vi "read device registers.vi"() -> (4 "Sorted Device Names":string[](array[string]), 6 "All Registers":T1(array[cluster]), 8 "Camera Registers":T1(array[cluster]), 15 "Found Registers":bool)   [LabVIEW 2010]
uses:
  <vilib>/Utility/file.llb/Read From Spreadsheet File (I64).vi
  <vilib>/Utility/file.llb/Read From Spreadsheet File (string).vi
panel:
  out "All registers":T2(array[cluster])
  in  "Register":T3
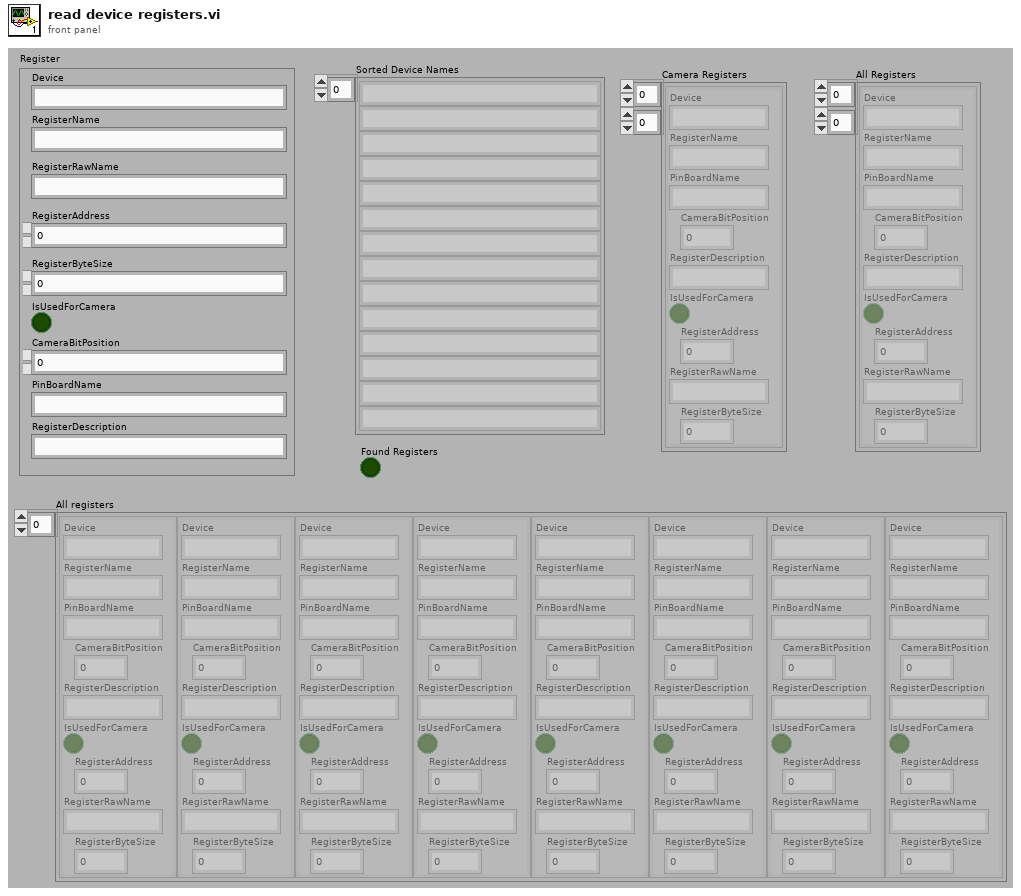
[diagram p1: front panel]
types:
  T1 = cluster{"Device":string, "RegisterName":string, "PinBoardName":string, "CameraBitPosition":i32, "RegisterDescription":string, "IsUsedForCamera":bool, "RegisterAddress":i32, "RegisterRawName":string, "RegisterByteSize":i32}[][]
  T2 = cluster{"Device":string, "RegisterName":string, "PinBoardName":string, "CameraBitPosition":i32, "RegisterDescription":string, "IsUsedForCamera":bool, "RegisterAddress":i32, "RegisterRawName":string, "RegisterByteSize":i32}[]
  T3 = cluster{"Device":string, "RegisterName":string, "PinBoardName":string, "CameraBitPosition":i32, "RegisterDescription":string, "IsUsedForCamera":bool, "RegisterAddress":i32, "RegisterRawName":string, "RegisterByteSize":i32}
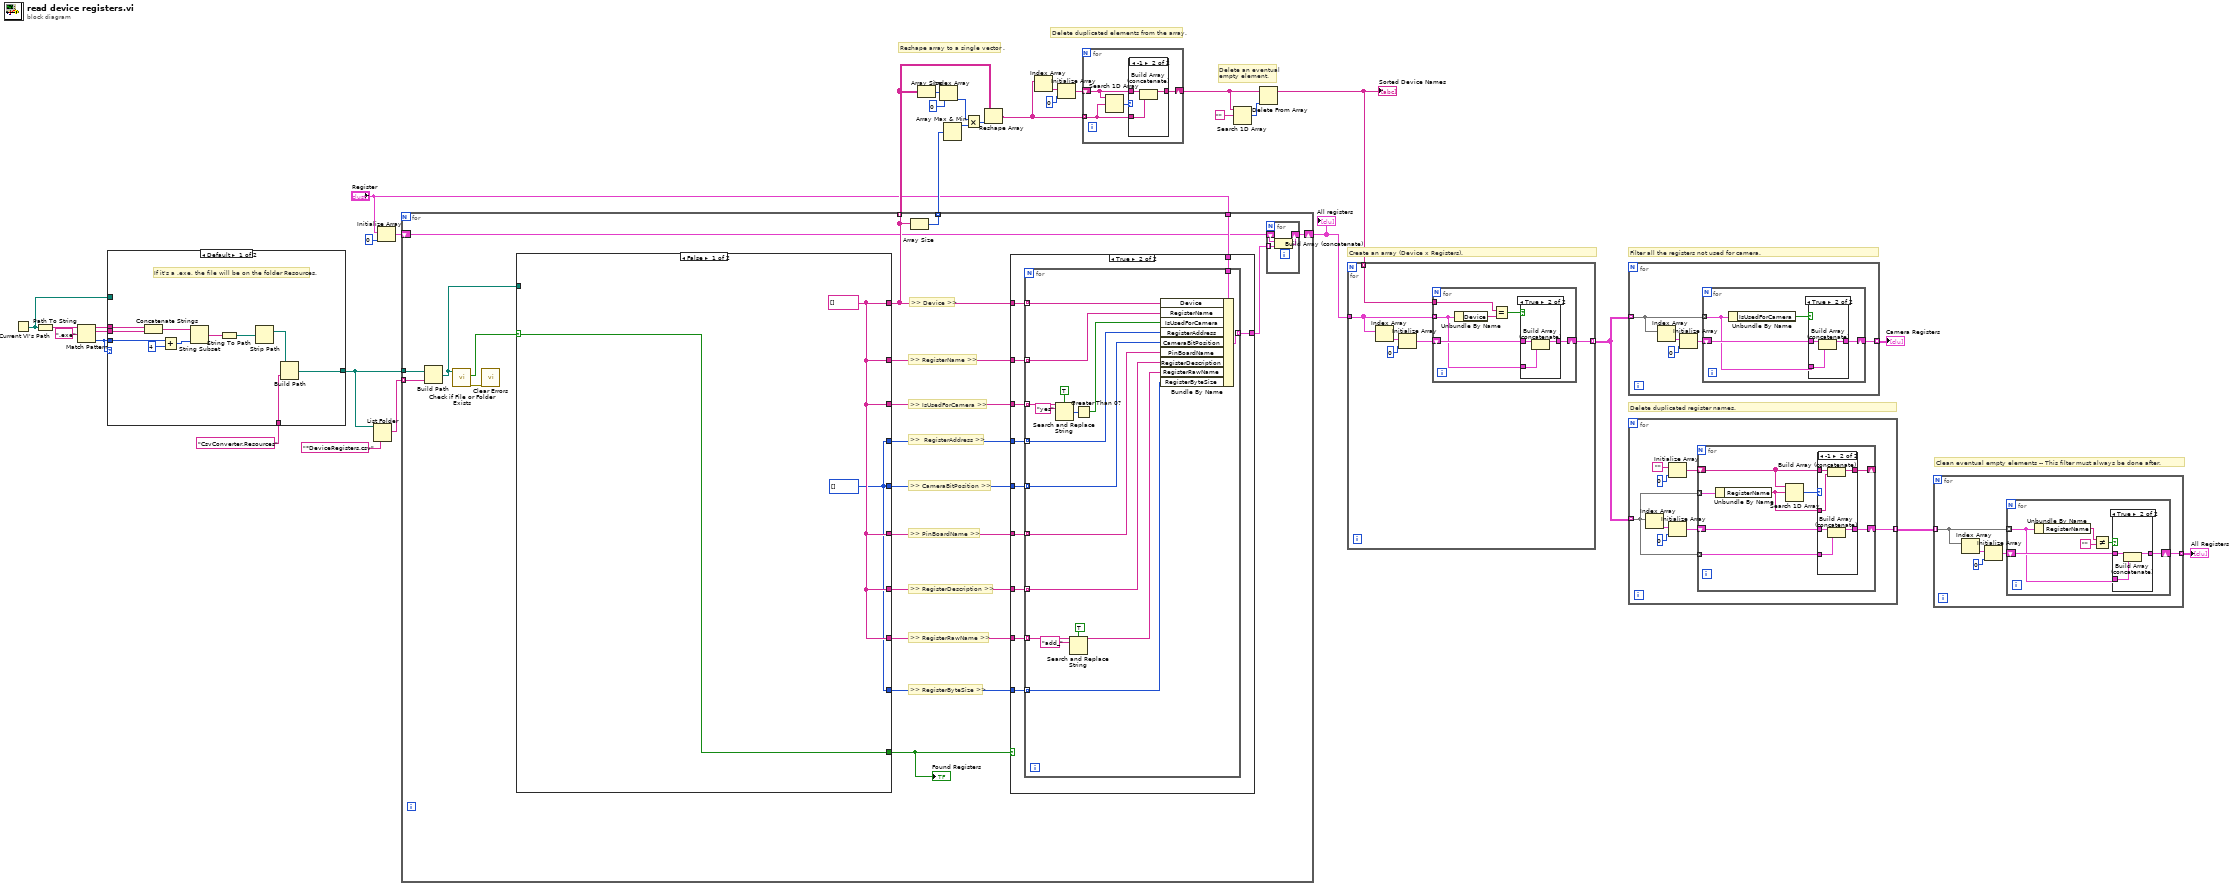
[diagram p0: block diagram]
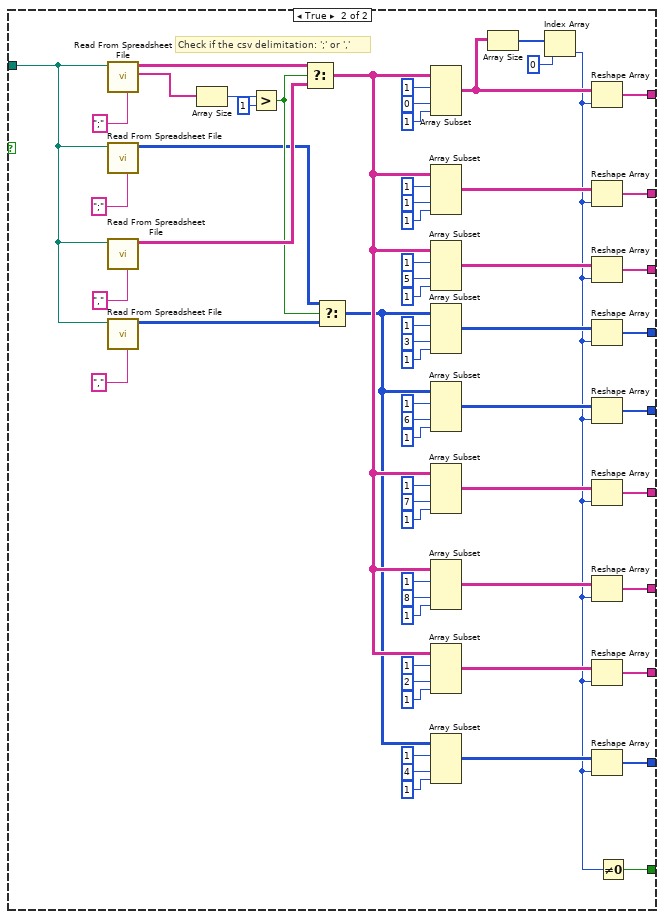
[diagram p8: hidden frame]
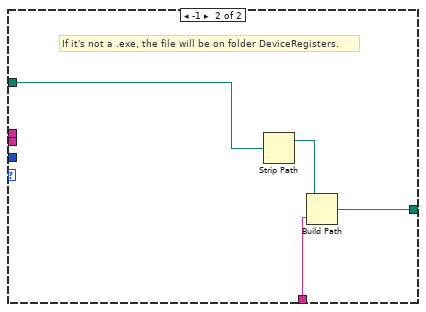
[diagram p9: hidden frame]
diagram:
  # "Clean eventual empty elements -- This filter must always be done after."
  # "Delete duplicated register names."
  # "Filter all the registers not used for camera."
  # "Create an array (Device x Registers)."
  # "Delete an eventual\nempty element."
  # "Delete duplicated elements from the array."
  # "Reshape array to a single vector ."
  n1 = Current VI's Path() -> (path=w28:path)
  n2 = Path To String(path=w28) -> (string=w33:string)
  n3 = Match Pattern(string=w33, regular expression=".exe") -> (before substring=w31:string, match substring=w30:string, offset past match=w29:i32)  [unwired: 1 in, 1 out]
  n4 = case shown="Default" w29 {
    tunnel: [w43 w46] -> w26
    tunnel: w31 -> [w42 _]
    tunnel: w30 -> [w41 _]
    tunnel: w29 -> [w39 _]
    tunnel: w28 -> [_ w47]
    tunnel: "CsvConverter.Resources" ("name or relative path") -> [w34 w45]
    frame Default {
      # "If it's a .exe, the file will be on the folder Resources."
      n5 = Concatenate Strings(w42, w41) -> (w40:string)
      n6 = Add(x=w39, y=4) -> (x+y=w38:i32)
      n7 = String Subset(string=w40, length (rest)=w38) -> (substring=w36:string)  [unwired: 1 in]
      n8 = String To Path(string=w36) -> (path=w35:path)
      n9 = Strip Path(path=w35) -> (stripped path=w44:path)  [unwired: 1 out]
      n10 = Build Path(base path=w44, name or relative path=w34) -> (appended path=w43:path)
    }
    frame -1 {
      # "If it's not a .exe, the file will be on folder DeviceRegisters."
      n11 = Strip Path(path=w47) -> (stripped path=w48:path)  [unwired: 1 out]
      n12 = Build Path(base path=w48, name or relative path=w45) -> (appended path=w46:path)
    }
  }
  n13 = List Folder(path=w26, pattern="*DeviceRegisters.csv") -> (filenames=w25:string[])  [unwired: 2 in, 3 out]
  n14 = Initialize Array("Register", 0 ("dimension size")) -> (w8:T2)
  n15 = for {
    tunnel: w26 -> [w66]
    tunnel: w25 -> [w64] mode=indexing
    tunnel: [w56] -> w23 mode=indexing
    tunnel: [w55] -> w24 mode=indexing
    shift-right: [w53] -> w6
    shift-left: w8 -> [w52]
    tunnel: "Register" -> [w54]
    # ">> RegisterByteSize >>"
    # ">> RegisterRawName >>"
    # ">> Device >>"
    # ">> RegisterName >>"
    # ">> IsUsedForCamera >>"
    # ">>  RegisterAddress >>"
    # ">> CameraBitPosition >>"
    # ">> RegisterDescription >>"
    # ">> PinBoardName >>"
    n16 = Build Path(base path=w66, name or relative path=w64) -> (appended path=w65:path)
    n17 = call <vilib>:"Check if File or Folder Exists.vi"("path"=w65) -> ("error out"=w68:errorcluster, "file or folder exists?"=w67:bool)  [unwired: 8 in, 1 out]
    n18 = call <vilib>:"Clear Errors.vi"("error in (no error)"=w68) -> ()  [unwired: 6 in, 1 out]
    n19 = case shown="False" w67 {
      selector: w67 -> [w103 _]
      tunnel: w65 -> [_ w163]
      tunnel: [w102 w142] -> w56
      tunnel: [w101 w139] -> w60
      tunnel: [w101 w138] -> w61
      tunnel: [w103 w137] -> w57
      tunnel: [w102 w136] -> w58
      tunnel: [w102 w127] -> w59
      tunnel: [w102 w126] -> w62
      tunnel: [w102 w119] -> w63
      tunnel: [w102 w115] -> w50
      tunnel: [w101 w104] -> w49
      frame False {
        w101 = i64[] []
        w102 = string[] []
      }
      frame True {
        # "Check if the csv delimitation: ';' or ','"
        n20 = call-poly <vilib>:"Read From Spreadsheet File.vi"("delimiter (\\t)"=";" ("delimiter (\\t)"), "file path (dialog if empty)"=w163) -> ("first row"=w160:string[], "all rows"=w159:string[][])  [unwired: 5 in, 3 out]
        n21 = call-poly <vilib>:"Read From Spreadsheet File.vi"("delimiter (\\t)"=";" ("delimiter (\\t)"), "file path (dialog if empty)"=w163) -> ("all rows"=w156:i64[][])  [unwired: 5 in, 4 out]
        n22 = call-poly <vilib>:"Read From Spreadsheet File.vi"("delimiter (\\t)"="," ("delimiter (\\t)"), "file path (dialog if empty)"=w163) -> ("all rows"=w158:string[][])  [unwired: 5 in, 4 out]
        n23 = call-poly <vilib>:"Read From Spreadsheet File.vi"("delimiter (\\t)"="," ("delimiter (\\t)"), "file path (dialog if empty)"=w163) -> ("all rows"=w155:i64[][])  [unwired: 5 in, 4 out]
        n24 = Array Size(array=w160) -> (size(s)=w162:i32)
        n25 = Greater?(x=w162, y=1) -> (0:w157:bool)
        n26 = Select(t=w159, s=w157, f=w158) -> (s? t:f=w107:string[][])
        n27 = Select(t=w156, s=w157, f=w155) -> (s? t:f=w105:i64[][])
        n28 = Array Subset(array=w107, index (row)=1 ("index"), index (col)=0 ("index"), length (col)=1 ("length")) -> (w143:string[][])  [unwired: 1 in]
        n29 = Array Subset(array=w107, index (row)=1 ("index"), index (col)=1 ("index"), length (col)=1 ("length")) -> (w135:string[][])  [unwired: 1 in]
        n30 = Array Subset(array=w107, index (row)=1 ("index"), index (col)=5 ("index"), length (col)=1 ("length")) -> (w128:string[][])  [unwired: 1 in]
        n31 = Array Subset(array=w105, index (row)=1 ("index"), index (col)=3 ("index"), length (col)=1 ("length")) -> (w141:i64[][])  [unwired: 1 in]
        n32 = Array Subset(array=w105, index (row)=1 ("index"), index (col)=6 ("index"), length (col)=1 ("length")) -> (w140:i64[][])  [unwired: 1 in]
        n33 = Array Subset(array=w107, index (row)=1 ("index"), index (col)=7 ("index"), length (col)=1 ("length")) -> (w125:string[][])  [unwired: 1 in]
        n34 = Array Subset(array=w107, index (row)=1 ("index"), index (col)=8 ("index"), length (col)=1 ("length")) -> (w120:string[][])  [unwired: 1 in]
        n35 = Array Subset(array=w107, index (row)=1 ("index"), index (col)=2 ("index"), length (col)=1 ("length")) -> (w114:string[][])  [unwired: 1 in]
        n36 = Array Subset(array=w105, index (row)=1 ("index"), index (col)=4 ("index"), length (col)=1 ("length")) -> (w110:i64[][])  [unwired: 1 in]
        n37 = Array Size(array=w143) -> (size(s)=w145:i32[])
        n38 = Index Array(array=w145, index=0) -> (element=w106:i32)
        n39 = Reshape Array(w143, w106) -> (w142:string[])
        n40 = Reshape Array(w135, w106) -> (w136:string[])
        n41 = Reshape Array(w128, w106) -> (w127:string[])
        n42 = Reshape Array(w141, w106) -> (w139:i64[])
        n43 = Reshape Array(w140, w106) -> (w138:i64[])
        n44 = Reshape Array(w125, w106) -> (w126:string[])
        n45 = Reshape Array(w120, w106) -> (w119:string[])
        n46 = Reshape Array(w114, w106) -> (w115:string[])
        n47 = Reshape Array(w110, w106) -> (w104:i64[])
        n48 = Not Equal To 0?(x=w106) -> (x != 0?=w137:bool)
      }
    }
    "Found Registers" <- w57
    n49 = Array Size(array=w56) -> (size(s)=w55:i32)
    n50 = case shown="True" w57 {
      tunnel: w63 -> [_ w82]
      tunnel: w62 -> [_ w81]
      tunnel: w61 -> [_ w80]
      tunnel: w60 -> [_ w79]
      tunnel: w59 -> [_ w78]
      tunnel: w58 -> [_ w77]
      tunnel: w56 -> [_ w76]
      tunnel: [_ w75] -> w51
      tunnel: w54 -> [_ w74]
      tunnel: w50 -> [_ w73]
      tunnel: w49 -> [_ w72]
      frame False {
      }
      frame True {
        n51 = for {
          tunnel: w82 -> [w90] mode=indexing
          tunnel: w81 -> [w91] mode=indexing
          tunnel: w80 -> [w92] mode=indexing
          tunnel: w79 -> [w93] mode=indexing
          tunnel: w78 -> [w100] mode=indexing
          tunnel: w77 -> [w95] mode=indexing
          tunnel: w76 -> [w94] mode=indexing
          tunnel: [w89] -> w75 mode=indexing
          tunnel: w74 -> [w88]
          tunnel: w73 -> [w86] mode=indexing
          tunnel: w72 -> [w83] mode=indexing
          n52 = Search and Replace String(case sensitive?=TRUE ("ignore case? (F)"), input string=w100, search string="yes") -> (number of replacements=w97:i32)  [unwired: 5 in, 3 out]
          n53 = Search and Replace String(case sensitive?=TRUE ("ignore case? (F)"), input string=w86, search string="add_") -> (result string=w87:string)  [unwired: 5 in, 3 out]
          n54 = Greater Than 0?(x=w97) -> (x > 0?=w96:bool)
          n55 = Bundle By Name(cluster=w88, "Device"=w94, "RegisterName"=w95, "IsUsedForCamera"=w96, "RegisterAddress"=w93, "CameraBitPosition"=w92, "PinBoardName"=w91, "RegisterDescription"=w90, "RegisterRawName"=w87, "RegisterByteSize"=w83) -> (w89:T3)
        }
      }
    }
    n56 = for {
      tunnel: w51 -> [w69] mode=indexing
      shift-right: [w71] -> w53
      shift-left: w52 -> [w70]
      n57 = Build Array (concatenate)(w70, w69) -> (w71:T2)
    }
  }
  "All registers" <- w6
  n58 = Array Size(array=w23) -> (size(s)=w21:i32[])
  n59 = Index Array(array=w21, index=0) -> (element=w18:i32)
  n60 = Array Max & Min(array=w24) -> (max value=w19:i32)  [unwired: 3 out]
  n61 = Multiply(x=w18, y=w19) -> (x*y=w20:i32)
  n62 = Reshape Array(w23, w20) -> (w14:string[])
  n63 = Index Array(array=w14) -> (element=w15:string)  [unwired: 1 in]
  n64 = Initialize Array(w15, 0 ("Dimension Size")) -> (w16:string[])
  n65 = for {
    tunnel: w14 -> [w170] mode=indexing
    shift-right: [w169] -> w12
    shift-left: w16 -> [w168]
    n66 = Search 1D Array(1D array=w168, element=w170) -> (index of element=w171:i32)  [unwired: 1 in]
    n67 = case shown="-1" w171 {
      tunnel: w170 -> [_ w175]
      tunnel: [w172 w173] -> w169
      tunnel: w168 -> [w172 w174]
      frame Default {
      }
      frame -1 {
        n68 = Build Array (concatenate)(w174, w175) -> (w173:string[])
      }
    }
  }
  n69 = Search 1D Array(1D array=w12, element="") -> (index of element=w11:i32)  [unwired: 1 in]
  n70 = Delete From Array(array=w12, index=w11) -> (array with subset deleted=w10:string[])  [unwired: 1 in, 1 out]
  "Sorted Device Names" <- w10
  n71 = for {
    tunnel: w10 -> [w181] mode=indexing
    tunnel: w6 -> [w178]
    tunnel: [w176] -> w5 mode=indexing
    n72 = Index Array(array=w178) -> (element=w180:T3)  [unwired: 1 in]
    n73 = Initialize Array(w180, 0 ("Dimension Size")) -> (w177:T2)
    n74 = for {
      tunnel: w181 -> [w184]
      tunnel: w178 -> [w182] mode=indexing
      shift-right: [w186] -> w176
      shift-left: w177 -> [w187]
      n75 = Unbundle By Name(w182) -> ("Device"=w185:string)
      n76 = Equal?(x=w184, y=w185) -> (x = y?=w183:bool)
      n77 = case shown="True" w183 {
        tunnel: [w188 w190] -> w186
        tunnel: w187 -> [w188 w191]
        tunnel: w182 -> [_ w189]
        frame False {
        }
        frame True {
          n78 = Build Array (concatenate)(w191, w189) -> (w190:T2)
        }
      }
    }
  }
  n79 = for {
    tunnel: w5 -> [w194] mode=indexing
    tunnel: [w192] -> w2 mode=indexing
    n80 = Index Array(array=w194) -> (element=w196:T3)  [unwired: 1 in]
    n81 = Initialize Array(w196, 0 ("Dimension Size")) -> (w193:T2)
    n82 = for {
      tunnel: w194 -> [w198] mode=indexing
      shift-right: [w199] -> w192
      shift-left: w193 -> [w200]
      n83 = Unbundle By Name(w198) -> ("IsUsedForCamera"=w197:bool)
      n84 = case shown="True" w197 {
        tunnel: [w201 w203] -> w199
        tunnel: w200 -> [w201 w204]
        tunnel: w198 -> [_ w202]
        frame False {
        }
        frame True {
          n85 = Build Array (concatenate)(w204, w202) -> (w203:T2)
        }
      }
    }
  }
  "Camera Registers" <- w2
  n86 = for {
    tunnel: w5 -> [w206] mode=indexing
    tunnel: [w205] -> w4 mode=indexing
    n87 = Index Array(array=w206) -> (element=w212:T3)  [unwired: 1 in]
    n88 = Initialize Array("", 0 ("Dimension Size")) -> (w207:string[])
    n89 = Initialize Array(w212, 0 ("Dimension Size")) -> (w211:T2)
    n90 = for {
      tunnel: w206 -> [w220] mode=indexing
      shift-right: [w219] -> w205
      shift-left: w211 -> [w218]
      shift-right: [w217] -> _
      shift-left: w207 -> [w216]
      tunnel: w206 -> [w215] mode=indexing
      n91 = Unbundle By Name(w215) -> ("RegisterName"=w213:string)
      n92 = Search 1D Array(1D array=w216, element=w213) -> (index of element=w214:i32)  [unwired: 1 in]
      n93 = case shown="-1" w214 {
        tunnel: w220 -> [_ w228]
        tunnel: [w222 w226] -> w219
        tunnel: w218 -> [w222 w227]
        tunnel: [w221 w224] -> w217
        tunnel: w216 -> [w221 w225]
        tunnel: w213 -> [_ w223]
        frame Default {
        }
        frame -1 {
          n94 = Build Array (concatenate)(w225, w223) -> (w224:string[])
          n95 = Build Array (concatenate)(w227, w228) -> (w226:T2)
        }
      }
    }
  }
  n96 = for {
    tunnel: w4 -> [w231] mode=indexing
    tunnel: [w229] -> w3 mode=indexing
    n97 = Index Array(array=w231) -> (element=w233:T3)  [unwired: 1 in]
    n98 = Initialize Array(w233, 0 ("Dimension Size")) -> (w230:T2)
    n99 = for {
      tunnel: w231 -> [w237] mode=indexing
      shift-right: [w238] -> w229
      shift-left: w230 -> [w239]
      n100 = Unbundle By Name(w237) -> ("RegisterName"=w235:string)
      n101 = Not Equal?(x=w235, y="") -> (x != y?=w234:bool)
      n102 = case shown="True" w234 {
        tunnel: [w240 w242] -> w238
        tunnel: w239 -> [w240 w243]
        tunnel: w237 -> [_ w241]
        frame False {
        }
        frame True {
          n103 = Build Array (concatenate)(w243, w241) -> (w242:T2)
        }
      }
    }
  }
  "All Registers" <- w3
